vi "remove last element_2Darray.vi"(11 "Input":dbl[][](array[numeric])) -> (3 "subarray":dbl[][](array[numeric]))   [LabVIEW 2023]
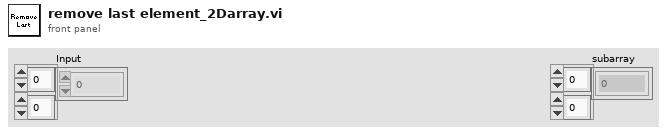
[diagram p1: front panel]
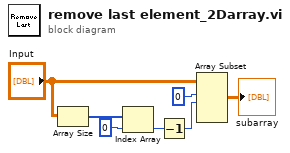
[diagram p0: block diagram]
diagram:
  n1 = Array Size(array="Input") -> (size(s)=w5:i32[])
  n2 = Index Array(array=w5, index=0) -> (element=w3:i32)
  n3 = Decrement(x=w3) -> (x-1=w1:i32)
  n4 = Array Subset(array="Input", index (row)=0 ("index"), length (row)=w1) -> (→"subarray":dbl[][])  [unwired: 2 in]
